vi "Open FPGA Refs and create P2P.vi"() -> (0 "error out":errorcluster, 1 "SlaveRef":T1, 2 "Master Ref":T2, 3 "P2P ref":refnum<k20>)   [LabVIEW 2015]
uses:
  Controls/FpgaMasterRef Typedef.ctl
  Controls/FpgaSlaveRef Typedef.ctl
  <vilib>/FPGAPlugInAG/PXIe-7972R/niLvFpga_Open_PXIe-7972R.vi
  <vilib>/FPGAPlugInAG/PXIe-7972R/niLvFpga_Abort_PXIe-7972R.vi
  <vilib>/Utility/error.llb/Error Cluster From Error Code.vi
  <vilib>/rvi/errors/niLvFpgaAdjustHostInterfaceError.vi
  <vilib>/rvi/interface/common/niFpgaWaitOnOcc.vi
  <vilib>/FPGAPlugInAG/PXIe-7972R/niLvFpga_Run_PXIe-7972R.vi
  <vilib>/rvi/interface/nirviOpenFPGA/nirviOpenFPGA.xnode
  FPGA Bitfiles/LidarMasterV5.1.4.lvbitx
  <vilib>/rvi/interface/nirviMethod/nirviMethod.xnode
  <vilib>/rvi/interface/nirviReadWriteControl/nirviReadWriteControl.xnode
  FPGA Bitfiles/LidarSlaveV5.1.4.lvbitx
  <vilib>/rvi/errors/niLvFpgaMergeErrorWithErrorCode.vi
  <vilib>/FPGAPlugInAG/PXIe-7972R/niLvFpga_P2PGetEndpoint_PXIe-7972R.vi
  NiFpgaLv.dll
  <vilib>/FPGAPlugInAG/PXIe-7972R/niLvFpga_ConfigureFifo_PXIe-7972R.vi
  <vilib>/FPGAPlugInAG/PXIe-7972R/niLvFpga_StartFifo_PXIe-7972R.vi
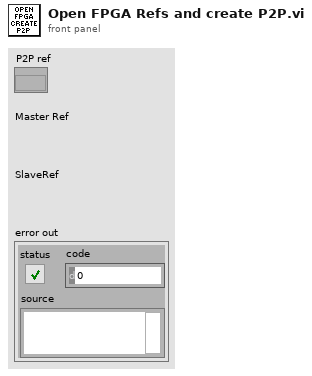
[diagram p1: front panel]
types:
  T1 = typedef "FpgaSlaveRef Typedef.ctl" = refnum<k20>
  T2 = typedef "FpgaMasterRef Typedef.ctl" = refnum<k20>
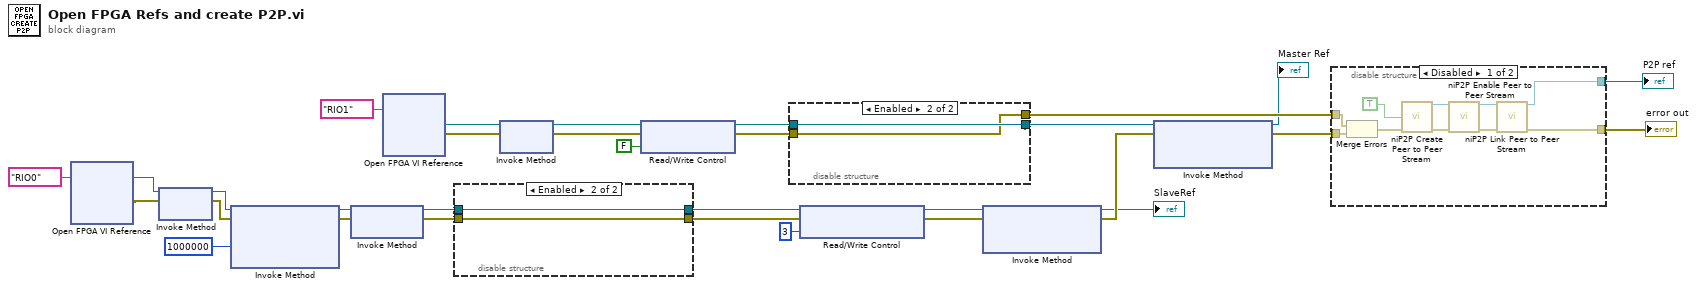
[diagram p0: block diagram]
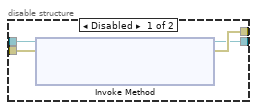
[diagram p3: hidden frame]
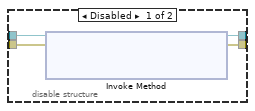
[diagram p4: hidden frame]
diagram:
  n1 = xnode "Open FPGA VI Reference"("resource name"=tag "RIO0") -> ("FPGA VI Reference Out"=w23:T1, "error out"=w24:errorcluster)  [unwired: 1 in]
  n2 = xnode "Invoke Method"("FPGA VI Reference In"=w23, "error in"=w24) -> ("FPGA VI Reference Out"=w25:T1, "error out"=w27:errorcluster)
  n3 = xnode "Invoke Method"("FPGA VI Reference In"=w25, "error in"=w27, "Requested Depth"=u32 1000000) -> ("FPGA VI Reference Out"=w28:T1, "error out"=w29:errorcluster)  [unwired: 1 out]
  n4 = xnode "Invoke Method"("FPGA VI Reference In"=w28, "error in"=w29) -> ("FPGA VI Reference Out"=w30:T1, "error out"=w31:errorcluster)
  n5 = xnode "Open FPGA VI Reference"("resource name"=tag "RIO1") -> ("FPGA VI Reference Out"=w21:T2, "error out"=w22:errorcluster)  [unwired: 1 in]
  n6 = disable-structure shown="Enabled" {
    disable-tunnel: w31 -> [w36 w37]
    disable-tunnel: w30 -> [w35 w38]
    disable-tunnel: [w33 w38] -> w13
    disable-tunnel: [w32 w37] -> w10
    frame Disabled {
      n7 = xnode "Invoke Method"("FPGA VI Reference In"=w35, "error in"=w36) -> ("FPGA VI Reference Out"=w33:T1, "error out"=w32:errorcluster, "Reader"=w34)
    }
    frame Enabled {
    }
  }
  n8 = xnode "Invoke Method"("FPGA VI Reference In"=w21, "error in"=w22) -> ("FPGA VI Reference Out"=w5:T2, "error out"=w3:errorcluster)
  n9 = xnode "Read/Write Control"("FPGA VI Reference In"=w5, "error in"=w3, "StartSyncLoop"=FALSE) -> ("FPGA VI Reference Out"=w4:T2, "error out"=w2:errorcluster)
  n10 = disable-structure shown="Enabled" {
    disable-tunnel: w2 -> [w43 w44]
    disable-tunnel: w4 -> [w42 w45]
    disable-tunnel: [w41 w44] -> w20
    disable-tunnel: [w40 w45] -> w15
    frame Disabled {
      n11 = xnode "Invoke Method"("FPGA VI Reference In"=w42, "error in"=w43) -> ("FPGA VI Reference Out"=w40:T2, "error out"=w41:errorcluster, "Writer"=w39)
    }
    frame Enabled {
    }
  }
  n12 = xnode "Read/Write Control"("FPGA VI Reference In"=w13, "error in"=w10, "Sample Clock Select"=u8 3) -> ("FPGA VI Reference Out"=w11:T1, "error out"=w9:errorcluster)
  n13 = xnode "Invoke Method"("FPGA VI Reference In"=w11, "error in"=w9) -> ("FPGA VI Reference Out"=→"SlaveRef":T1, "error out"=w16:errorcluster)  [unwired: 1 in]
  n14 = xnode "Invoke Method"("FPGA VI Reference In"=w15, "error in"=w16) -> ("FPGA VI Reference Out"=→"Master Ref":T2, "error out"=w19:errorcluster)  [unwired: 1 in]
  n15 = disable-structure shown="Disabled" {
    disable-tunnel: w20 -> [w57 _]
    disable-tunnel: w19 -> [w56 w58]
    disable-tunnel: [w54 w58] -> w17
    disable-tunnel: [w53 _] -> w14
    frame Disabled {
      n16 = Merge Errors(w57, w56) -> (w55:errorcluster)
      n17 = call <vilib>:"niP2P Create Peer to Peer Stream.vi"("enable stream (T)"=TRUE, "error in (no error)"=w55) -> ("writer"=w46:refnum<k20>, "stream session"=w49:refnum<k20>, "reader"=w47:refnum<k20>, "error out"=w50:errorcluster)  [unwired: 10 in]
      n18 = call <vilib>:"niP2P Enable Peer to Peer Stream.vi"("stream session"=w49, "error in (no error)"=w50) -> ("stream session out"=w51:refnum<k20>, "error out"=w52:errorcluster)  [unwired: 12 in]
      n19 = call <vilib>:"niP2P Link Peer to Peer Stream.vi"("stream session"=w51, "error in (no error)"=w52) -> ("stream session out"=w53:refnum<k20>, "error out"=w54:errorcluster)  [unwired: 12 in]
    }
    frame Enabled {
    }
  }
  "error out" <- w17
  "P2P ref" <- w14
